vi "TCP Connection Manager.vi"(6 "properties in":T1, 8 "error in":errorcluster, 9 "method":T4, 10 "index":i32, 11 "connection in":T2) -> (0 "error out":errorcluster, 1 "number of connections":i32, 2 "all connections":T2[](array[typedef]), 3 "connection out":T2, 4 "properties out":T1, 5 "all properties":T1[](array[typedef]))   [LabVIEW 2010, in "NI STM.lvlib"]
doc: "This VI maintains the list of host connections. \n\nCopyright 2015, 2016, 2017 National Instruments Corporation\n\nLicensed under the Apache License, Version 2.0 (the \"License\"); you may not use this file except in compliance with the License.\n\n You may obtain a copy of the License at\n\n http://www.apache.org/licenses/LICENSE-2.0\n\nUnless required by applicable law or agreed to in writing, software distributed under the License is distributed on an \"AS IS\" BASIS, WITHOUT WARRANTIES OR CONDITIONS OF ANY KIND, either express or implied.\n\nSee the License for the specific language governing permissions and limitations under the License."
uses:
  NI STM.lvlib
  TCP Connection Method.ctl
  TCP/TCP Connection Info.ctl
  SubVIs/MetaDataElement.ctl
  TCP Connection Properties.ctl
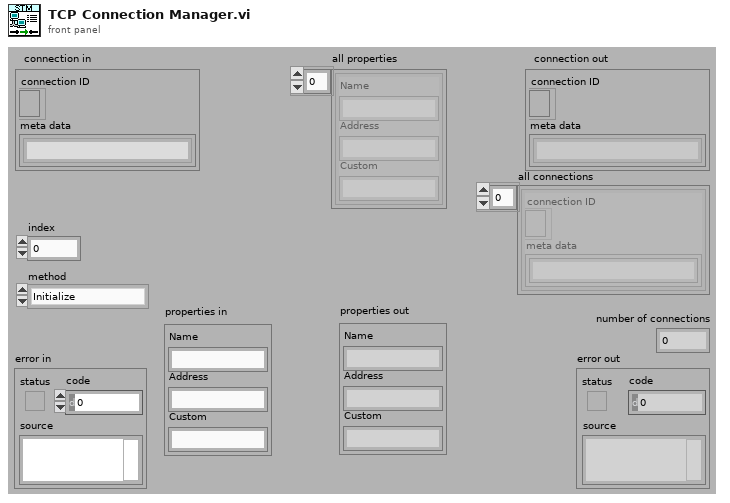
[diagram p1: front panel]
types:
  T1 = typedef "NI STM.lvlib/TCP Connection Properties.ctl" = cluster{"Name":string, "Address":string, "Custom":string}
  T2 = typedef "NI STM.lvlib/TCP Connection Info.ctl" = cluster{"connection ID":refnum<k5>, "meta data":T3[]}
  T3 = typedef "NI STM.lvlib/MetaDataElement.ctl" = string
  T4 = typedef "NI STM.lvlib/TCP Connection Method.ctl" = enum16{"Initialize", "Add Connection", "Set Properties", "Get Connection(s)", "Remove Connection", "Remove All Connections", "Get Connection Count"}
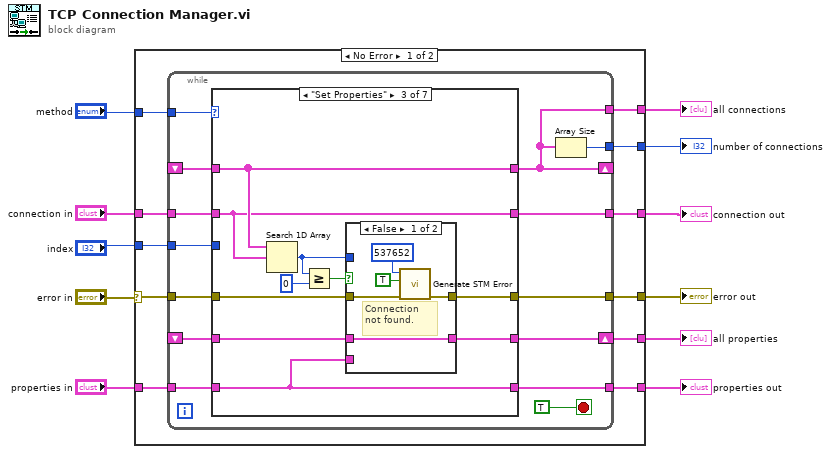
[diagram p0: block diagram]
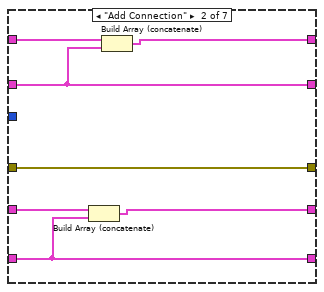
[diagram p3: hidden frame]
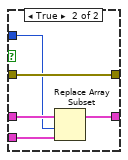
[diagram p4: hidden frame]
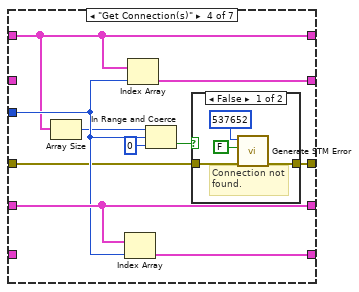
[diagram p5: hidden frame]
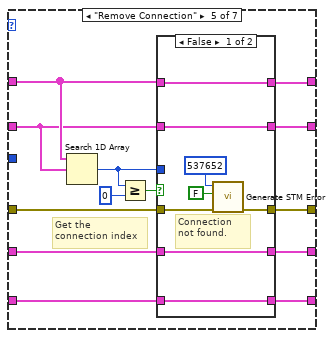
[diagram p7: hidden frame]
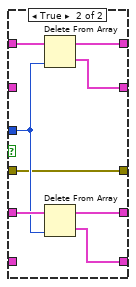
[diagram p8: hidden frame]
diagram:
  n1 = case shown="No Error" "error in" {
    selector: "error in" -> [w22 w116]
    tunnel: [w21 w116] -> w10
    tunnel: "index" -> [w20 _]
    tunnel: "method" -> [w19 _]
    tunnel: "connection in" -> [w18 w115]
    tunnel: [w17 _] -> w6
    tunnel: [w16 _] -> w5
    tunnel: [w15 w115] -> w4
    tunnel: "properties in" -> [w14 _]
    tunnel: [w13 _] -> w2
    tunnel: [w12 _] -> w1
    frame No Error {
      n2 = while {
        shift-right: [w28] -> _
        shift-left: _ -> [w35]
        tunnel: w22 -> [w34]
        tunnel: [w33] -> w21
        tunnel: w20 -> [w32]
        tunnel: w19 -> [w31]
        tunnel: w18 -> [w30]
        tunnel: [w29] -> w17
        tunnel: [w28] -> w16
        tunnel: [w27] -> w15
        shift-right: [w24] -> w13
        shift-left: _ -> [w26]
        tunnel: w14 -> [w25]
        tunnel: [w23] -> w12
        stop <- TRUE stop-if-true
        n3 = case shown="\"Set Properties\"" w31 {
          tunnel: w35 -> [_ w44 w53 w70 w92 _ w114]
          tunnel: w30 -> [_ w42 w52 _ w84 _ w113]
          tunnel: [_ w43 w53 w70 w88 _ w114] -> w28
          tunnel: [_ w42 w52 w74 w87 _ w113] -> w27
          tunnel: [w37 w41 w49 w65 w86 w109 w112] -> w33
          tunnel: w34 -> [w37 w41 w50 w68 w85 w109 w112]
          tunnel: w32 -> [_ _ _ w71 _ _ _]
          tunnel: w26 -> [_ w40 w48 w73 w83 _ w111]
          tunnel: w25 -> [_ w38 w45 _ w80 _ w110]
          tunnel: [_ w39 w46 w73 w82 _ w111] -> w24
          tunnel: [_ w38 w45 w72 w81 _ w110] -> w23
          frame "Initialize" {
          }
          frame "Add Connection" {
            n4 = Build Array (concatenate)(w40, w38) -> (w39:T1[])
            n5 = Build Array (concatenate)(w44, w42) -> (w43:T2[])
          }
          frame "Set Properties" {
            n6 = Search 1D Array(1D array=w53, element=w52) -> (index of element=w47:i32)  [unwired: 1 out]
            n7 = Greater Or Equal?(x=w47, y=0) -> (x >= y?=w51:bool)
            n8 = case shown="False" w51 {
              tunnel: w50 -> [w56 w64]
              tunnel: [w55 w64] -> w49
              tunnel: w48 -> [w59 w63]
              tunnel: w47 -> [_ w62]
              tunnel: w45 -> [_ w61]
              tunnel: [w59 w60] -> w46
              frame False {
                # "Connection not found."
                n9 = call "Generate STM Error.vi"("error in"=w56, "status (T)"=TRUE, "code"=537652) -> ("error out"=w55:errorcluster)  [unwired: 8 in]
              }
              frame True {
                n10 = Replace Array Subset(array=w63, new element=w61, index=w62) -> (w60:T1[])
              }
            }
          }
          frame "Get Connection(s)" {
            n11 = Array Size(array=w70) -> (size(s)=w69:i32)
            n12 = Index Array(array=w73, index=w71) -> (element=w72:T1)
            n13 = Index Array(array=w70, index=w71) -> (element=w74:T2)
            n14 = In Range and Coerce(upper limit=w69, x=w71, lower limit=0) -> (In Range?=w67:bool)  [unwired: 1 out]
            n15 = case shown="False" w67 {
              tunnel: w68 -> [w76 w79]
              tunnel: [w75 w79] -> w65
              frame False {
                # "Connection not found."
                n16 = call "Generate STM Error.vi"("error in"=w76, "status (T)"=FALSE, "code"=537652) -> ("error out"=w75:errorcluster)  [unwired: 8 in]
              }
              frame True {
              }
            }
          }
          frame "Remove Connection" {
            # "Get the \nconnection index"
            n17 = Search 1D Array(1D array=w92, element=w84) -> (index of element=w91:i32)  [unwired: 1 out]
            n18 = Greater Or Equal?(x=w91, y=0) -> (x >= y?=w89:bool)
            n19 = case shown="False" w89 {
              tunnel: w92 -> [w100 w107]
              tunnel: w91 -> [_ w104]
              tunnel: [w100 w108] -> w88
              tunnel: [w99 w102] -> w87
              tunnel: [w93 w101] -> w86
              tunnel: w85 -> [w94 w101]
              tunnel: w84 -> [w99 _]
              tunnel: w83 -> [w98 w106]
              tunnel: [w98 w105] -> w82
              tunnel: [w97 w103] -> w81
              tunnel: w80 -> [w97 _]
              frame False {
                # "Connection not found."
                n20 = call "Generate STM Error.vi"("error in"=w94, "status (T)"=FALSE, "code"=537652) -> ("error out"=w93:errorcluster)  [unwired: 8 in]
              }
              frame True {
                n21 = Delete From Array(array=w107, index=w104) -> (deleted portion=w102:T2, array with subset deleted=w108:T2[])  [unwired: 1 in]
                n22 = Delete From Array(array=w106, index=w104) -> (deleted portion=w103:T1, array with subset deleted=w105:T1[])  [unwired: 1 in]
              }
            }
          }
          frame "Remove All Connections" {
          }
          frame "Get Connection Count" {
          }
        }
        n23 = Array Size(array=w28) -> (size(s)=w29:i32)
      }
    }
    frame Error {
    }
  }
  "error out" <- w10
  "number of connections" <- w6
  "all connections" <- w5
  "connection out" <- w4
  "all properties" <- w2
  "properties out" <- w1
